vi "Facade.vi"(0 "Data In":T5, 2 "Display State In":T3, 3 "Container State":T4) -> (6 "Data Out":T5, 7 "Display State Out":T3, 8 "Action":T2)   [LabVIEW 2015, in "Level.xctl"]
uses:
  Level.xctl
  Data.vi
  Classes/Level/Level.lvclass
  <vilib>/_xctls/Container State.ctl
  State.vi
  <vilib>/_xctls/Action.ctl
  Classes/Level/LevelUnits.ctl
  Classes/Level/Level.lvclass/Level.ctl
  Classes/Level/Read Level.vi
  Classes/Level/Read Units.vi
  Classes/Level/Read Spectrum Level.vi
  Classes/Level/Read max.vi
  Classes/Level/Write Level.vi
  Classes/Level/Write Units.vi
  Classes/Level/Write Spectrum Level.vi
  <vilib>/_xctls/XControlSupport.lvlib
panel:
  in  "Units Enum":T1
  in  "Spectrum level":bool
  in  "Units":u16(ring)
  out "Max":dbl
  in  "Level":dbl
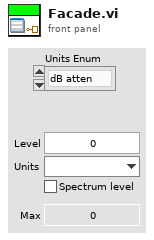
[diagram p1: front panel]
types:
  T1 = typedef "Level.lvclass/LevelUnits.ctl" = enum16{"dB atten", "dB SPL", "dB Vrms", "Volts", "dB mW", "mW", "dB HL", "dB SL"}
  T2 = typedef "XControlSupport.lvlib/Action.ctl" = cluster{"Data Changed?":bool, "State Changed?":bool, "Action Name":string}
  T3 = typedef "Level.xctl/State.vi" = cluster{"action":string, "excluded":enum16{"dB Atten", "dB Vrms", "dB SPL"}[]}
  T4 = typedef "XControlSupport.lvlib/Container State.ctl" = cluster{"Indicator?":bool, "Run Mode?":bool, " Refnum":refnum<vi>}
  T5 = typedef "Level.xctl/Data.vi" = refnum<class "Level.lvclass">
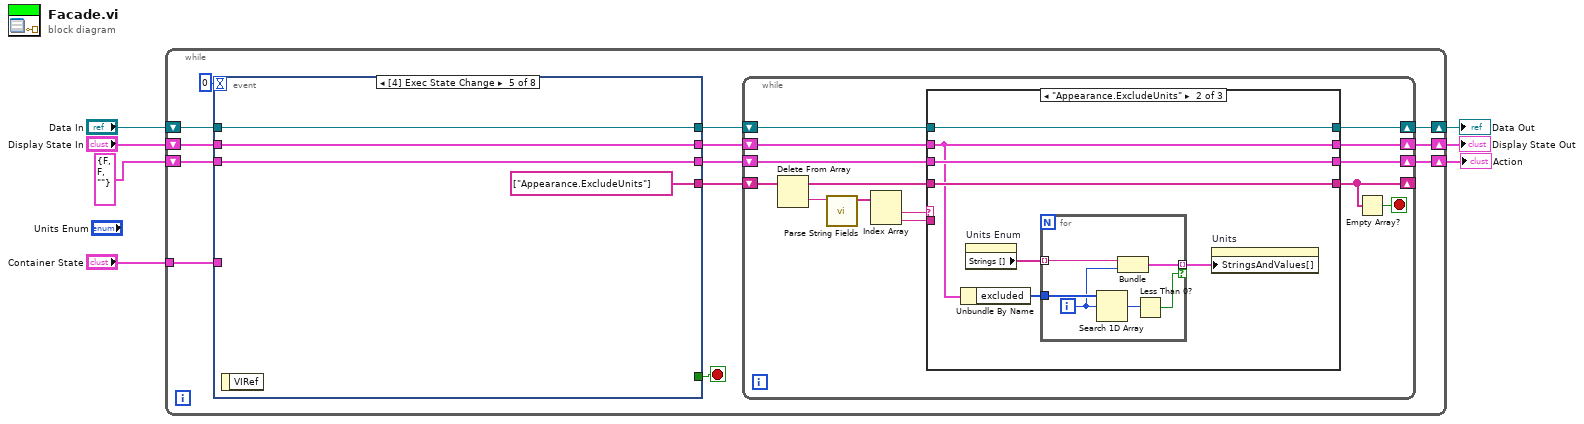
[diagram p0: block diagram]
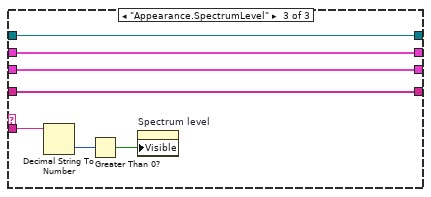
[diagram p3: hidden frame]
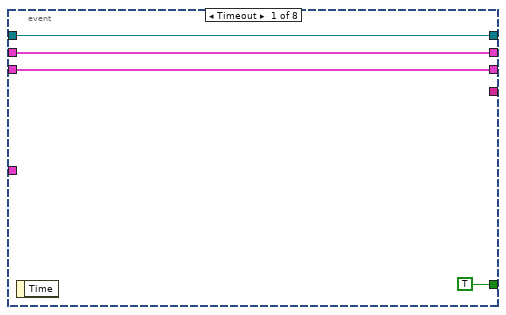
[diagram p4: hidden frame]
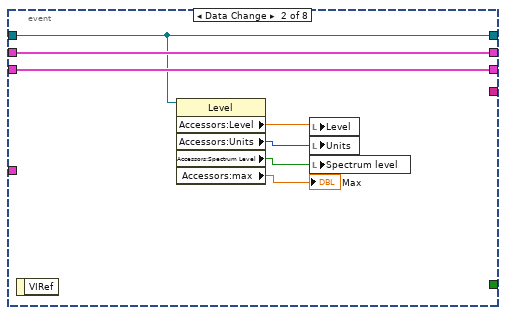
[diagram p5: hidden frame]
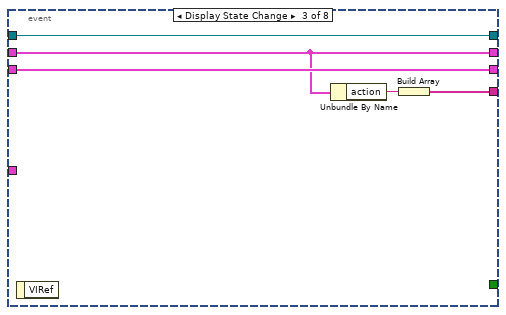
[diagram p6: hidden frame]
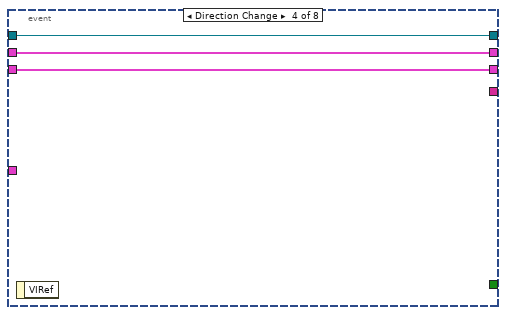
[diagram p7: hidden frame]
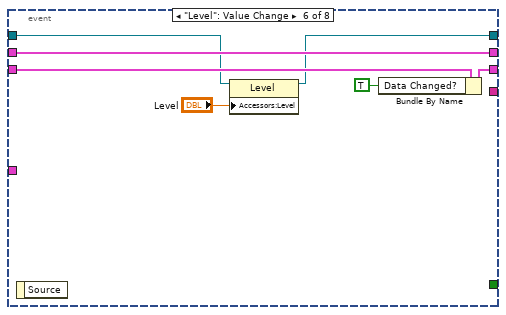
[diagram p8: hidden frame]
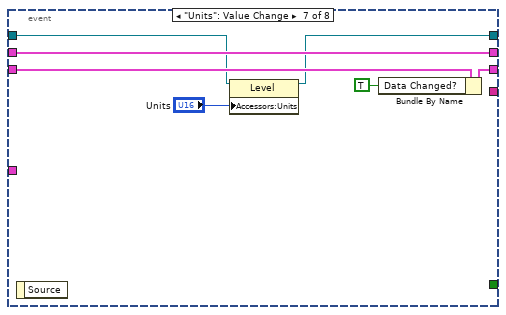
[diagram p9: hidden frame]
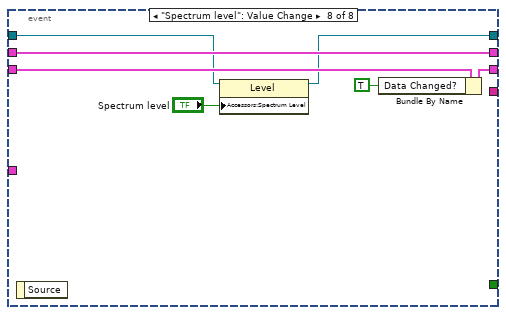
[diagram p10: hidden frame]
diagram:
  n1 = while {
    shift-right: [w9] -> w4
    shift-left: "Display State In" -> [w20]
    tunnel: "Container State" -> [w17]
    shift-right: [w10] -> w7
    shift-left: "Data In" -> [w16]
    shift-right: [w8] -> w2
    shift-left: T2 {"Data Changed?"=FALSE, "State Changed?"=FALSE, "Action Name"=""} ("Action") -> [w15]
    stop <- w19 stop-if-true
    n2 = event shown="[4] Exec State Change" {
      selector: _ -> [_ _ _ _ _ _ _ _]
      dyn-events: _ -> [_ _ _ _ _ _ _ _]
      timeout: 0 -> [_ _ _ _ _ _ _ _]
      tunnel: w20 -> [w60 w69 w72 w77 w81 w88 w95 w102]
      tunnel: [w60 w69 w72 w77 w81 w88 w95 w102] -> w12
      tunnel: [TRUE _ _ _ _ _ _ _] -> w19
      tunnel: w17 -> [_ _ _ _ _ _ _ _]
      tunnel: w16 -> [w59 w67 w74 w76 w80 w84 w91 w98]
      tunnel: [w59 w67 w74 w76 w80 w83 w90 w97] -> w13
      tunnel: [w61 w68 w73 w75 w79 w86 w93 w100] -> w11
      tunnel: w15 -> [w61 w68 w73 w75 w79 w87 w94 w101]
      tunnel: [_ _ w70 _ string[] ["Appearance.ExcludeUnits"] _ _ _] -> w14
      event Timeout {
        n3 = event-data() -> ()  [unwired: 1 in, 1 out]
      }
      event Data Change {
        n4 = event-data() -> ()  [unwired: 1 in, 1 out]
        n5 = property class="Level"(reference=w67) -> ("Accessors:Level"=w65:dbl, "Accessors:Units"=w64:T1, "Accessors:Spectrum Level"=w63:bool, "Accessors:max"=→"Max":dbl)  [unwired: 1 in, 2 out]
        n6 = local write "Level"(w65) -> ()
        n7 = local write "Units"(w64) -> ()
        n8 = local write "Spectrum level"(w63) -> ()
      }
      event Display State Change {
        n9 = event-data() -> ()  [unwired: 1 in, 1 out]
        n10 = Unbundle By Name(w72) -> ("action"=w71:string)
        n11 = Build Array(w71) -> (w70:string[])
      }
      event Direction Change {
        n12 = event-data() -> ()  [unwired: 1 in, 1 out]
      }
      event Exec State Change {
        n13 = event-data() -> ()  [unwired: 1 in, 1 out]
      }
      event "Level": Value Change {
        n14 = event-data() -> ()  [unwired: 1 in, 1 out]
        n15 = property class="Level"(reference=w84, "Accessors:Level"="Level") -> (reference out=w83:T5)  [unwired: 1 in, 1 out]
        n16 = Bundle By Name(cluster=w87, "Data Changed?"=TRUE) -> (w86:T2)
      }
      event "Units": Value Change {
        n17 = event-data() -> ()  [unwired: 1 in, 1 out]
        n18 = property class="Level"(reference=w91, "Accessors:Units"="Units") -> (reference out=w90:T5)  [unwired: 1 in, 1 out]
        n19 = Bundle By Name(cluster=w94, "Data Changed?"=TRUE) -> (w93:T2)
      }
      event "Spectrum level": Value Change {
        n20 = event-data() -> ()  [unwired: 1 in, 1 out]
        n21 = property class="Level"(reference=w98, "Accessors:Spectrum Level"="Spectrum level") -> (reference out=w97:T5)  [unwired: 1 in, 1 out]
        n22 = Bundle By Name(cluster=w101, "Data Changed?"=TRUE) -> (w100:T2)
      }
    }
    n23 = while {
      shift-right: [w32] -> _
      shift-left: w14 -> [w34]
      shift-right: [w25] -> w8
      shift-left: w11 -> [w28]
      shift-right: [w26] -> w9
      shift-left: w12 -> [w29]
      shift-right: [w27] -> w10
      shift-left: w13 -> [w30]
      stop <- w31 stop-if-true
      n24 = Delete From Array(array=w34) -> (deleted portion=w24:string, array with subset deleted=w33:string[])  [unwired: 2 in]
      n25 = call "Parse String Fields.vi"("String"=w24) -> ("Fields"=w23:string[])  [unwired: 9 in, 1 out]
      n26 = Index Array(array=w23) -> (element #1=w22:string, element #2=w21:string)  [unwired: 2 in]
      n27 = case shown="\"Appearance.ExcludeUnits\"" w22 {
        tunnel: w33 -> [w38 w45 w58]
        tunnel: [w38 w45 w58] -> w32
        tunnel: w30 -> [w37 w44 w57]
        tunnel: w29 -> [w36 w41 w56]
        tunnel: w28 -> [w35 w43 w55]
        tunnel: [w37 w44 w57] -> w27
        tunnel: [w36 w41 w56] -> w26
        tunnel: [w35 w43 w55] -> w25
        tunnel: w21 -> [_ _ w53]
        frame "", Default {
        }
        frame "Appearance.ExcludeUnits" {
          n28 = Unbundle By Name(w41) -> ("excluded"=w39:enum16{"dB Atten", "dB Vrms", "dB SPL"}[])
          n29 = property on="Units Enum" class="Enum (strict)"() -> ("Strings []"=w42:string[])  [unwired: 2 in, 2 out]
          n30 = for {
            tunnel: w42 -> [w51] mode=indexing
            tunnel: [w50] -> w40 mode=indexing if=w46
            tunnel: w39 -> [w49]
            i -> [w48]
            n31 = Search 1D Array(1D array=w49, element=w48) -> (index of element=w47:i32)  [unwired: 1 in]
            n32 = Bundle(w51, w48) -> (w50:cluster{string, i32})  [unwired: 1 in]
            n33 = Less Than 0?(x=w47) -> (x < 0?=w46:bool)
          }
          n34 = property on="Units" class="Ring (strict)"("StringsAndValues[]"=w40) -> ()  [unwired: 2 in, 2 out]
        }
        frame "Appearance.SpectrumLevel" {
          n35 = Decimal String To Number(string=w53) -> (number=w54:i32)  [unwired: 2 in, 1 out]
          n36 = Greater Than 0?(x=w54) -> (x > 0?=w52:bool)
          n37 = property on="Spectrum level" class="Bool (strict)"("Visible"=w52) -> ()  [unwired: 2 in, 2 out]
        }
      }
      n38 = Empty Array?(array=w32) -> (empty?=w31:bool)
    }
  }
  "Display State Out" <- w4
  "Data Out" <- w7
  "Action" <- w2
